vi "Three part tester.vi"() -> ()   [LabVIEW 2009]
uses:
  <vilib>/Instr/_visa.llb/VISA Configure Serial Port (Instr).vi
panel:
  out "Cluster Display":T1
  out "Cluster 2 Display":T2
  in  "Stop":bool
  out "decimal integer string 2":string
  out "number 2":u8 format="%b"
  in  "Yellow Guitar LED":bool
  in  "Green Guitar LED":bool
  in  "Red Guitar LED":bool
  in  "Blue Guitar LED":bool
  in  "Orange Guitar LED":bool
  in  "Orange Bass LED":bool
  in  "Yellow Bass LED":bool
  in  "Green Bass LED":bool
  in  "Red Bass LED":bool
  in  "Blue Bass LED":bool
  in  "Red Drum":bool
  in  "GreenDrum":bool
  in  "VISA resource name":refnum<visa-resource-name>
  out "number":u8 format="%b"
  out "decimal integer string":string
  in  "Yellow Drum":bool
  in  "Blue Drum":bool
  # "Drums"
  # "Bass"
  # "Guitar"
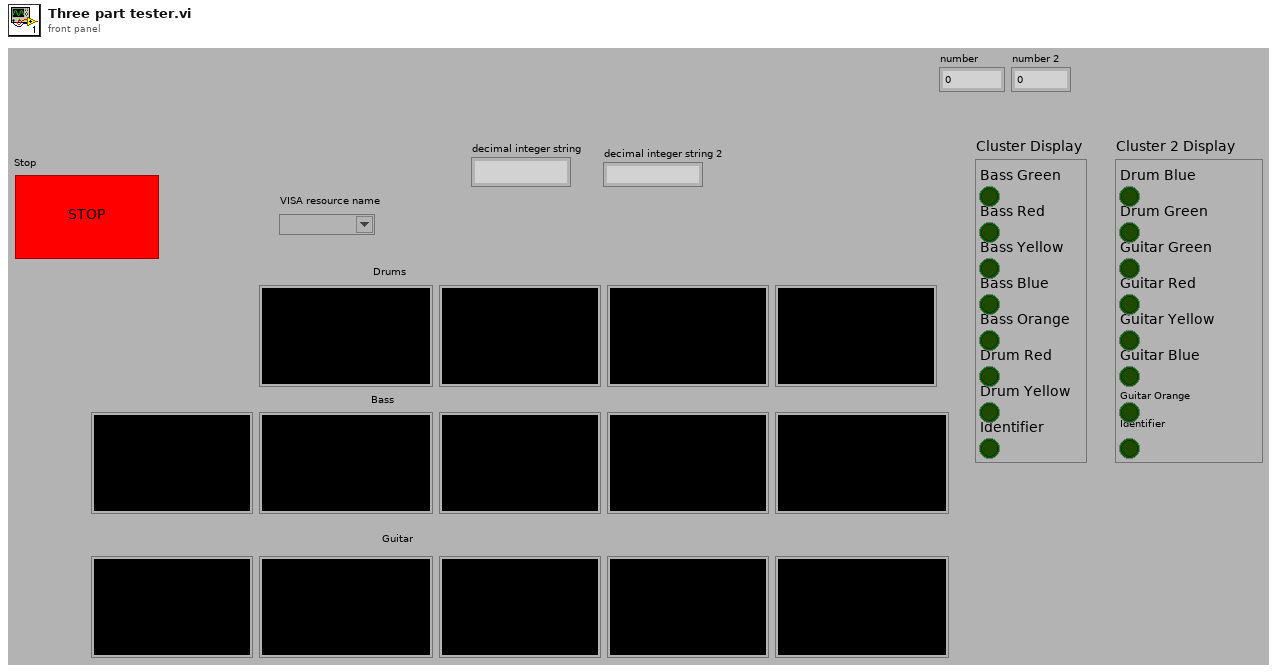
[diagram p1: front panel]
types:
  T1 = cluster{"Bass Green":bool, "Bass Red":bool, "Bass Yellow":bool, "Bass Blue":bool, "Bass Orange":bool, "Drum Red":bool, "Drum Yellow ":bool, "Identifier":bool}
  T2 = cluster{"Drum Blue":bool, "Drum Green":bool, "Guitar Green":bool, "Guitar Red":bool, "Guitar Yellow":bool, "Guitar Blue":bool, "Guitar Orange":bool, "Identifier":bool}
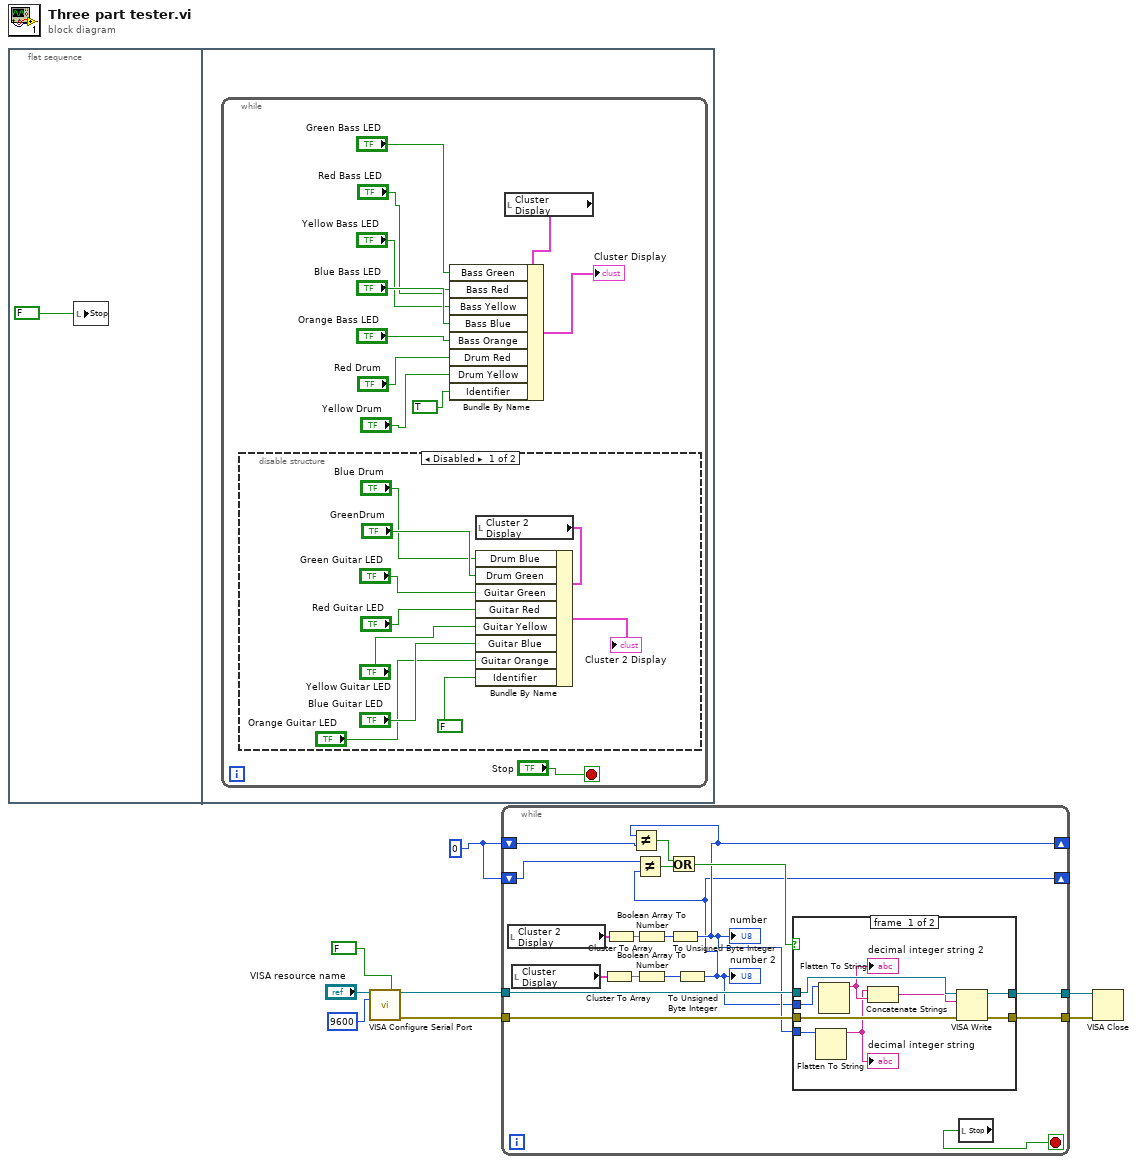
[diagram p0: block diagram]
diagram:
  w1 = u8 0
  n1 = flat-sequence {
    frame #0 {
      n2 = local write "Stop"(FALSE ("Stop 2")) -> ()
    }
    frame #1 {
      n3 = while {
        stop <- "Stop" stop-if-true
        n4 = disable-structure shown="Disabled" {
          frame #0 {
            n5 = local read "Cluster 2 Display"() -> (w29:T2)
            n6 = Bundle By Name(cluster=w29, "Drum Blue"="Blue Drum", "Drum Green"="GreenDrum", "Guitar Green"="Green Guitar LED", "Guitar Red"="Red Guitar LED", "Guitar Yellow"="Yellow Guitar LED", "Guitar Blue"="Blue Guitar LED", "Guitar Orange"="Orange Guitar LED", "Identifier"=FALSE ("element")) -> (→"Cluster 2 Display":T2)
          }
          frame #1 {
          }
        }
        n7 = local read "Cluster Display"() -> (w19:T1)
        n8 = Bundle By Name(cluster=w19, "Bass Green"="Green Bass LED", "Bass Red"="Red Bass LED", "Bass Yellow"="Yellow Bass LED", "Bass Blue"="Blue Bass LED", "Bass Orange"="Orange Bass LED", "Drum Red"="Red Drum", "Drum Yellow"="Yellow Drum", "Identifier"=TRUE ("element")) -> (→"Cluster Display":T1)
      }
    }
  }
  n9 = call-poly "VISA Configure Serial Port"("VISA resource name"="VISA resource name", "Enable Termination\nChar (T)"=FALSE ("Enable Termination\nChar (T)"), "baud rate (9600)"=u32 9600) -> ("VISA resource name out"=w8:refnum<visa-resource-name>, "error out"=w3:errorcluster)  [unwired: 11 in]
  n10 = while {
    tunnel: w8 -> [w48]
    tunnel: [w47] -> w7
    tunnel: w3 -> [w46]
    tunnel: [w45] -> w2
    shift-right: [w34] -> _
    shift-left: w1 -> [w33]
    shift-right: [w32] -> _
    shift-left: w1 -> [w31]
    stop <- w40 stop-if-true
    n11 = local read "Cluster 2 Display"() -> (w41:T2)
    n12 = local read "Cluster Display"() -> (w42:T1)
    n13 = Cluster To Array(cluster=w42) -> (array=w43:bool[])
    n14 = Cluster To Array(cluster=w41) -> (array=w44:bool[])
    n15 = Boolean Array To Number(Boolean array=w44) -> (number=w39:u32)
    n16 = Boolean Array To Number(Boolean array=w43) -> (number=w38:u32)
    n17 = To Unsigned Byte Integer(number=w39) -> (unsigned 8bit integer=w34:u8)
    "number" <- w34
    n18 = Not Equal?(x=w34, y=w33) -> (x != y?=w36:bool)
    n19 = To Unsigned Byte Integer(number=w38) -> (unsigned 8bit integer=w32:u8)
    "number 2" <- w32
    n20 = Not Equal?(x=w31, y=w32) -> (x != y?=w37:bool)
    n21 = Or(x=w36, y=w37) -> (x .or. y?=w35:bool)
    n22 = case shown="False" w35 {
      tunnel: w48 -> [w57 w59]
      tunnel: [w56 w59] -> w47
      tunnel: w34 -> [w50 _]
      tunnel: w46 -> [w55 w58]
      tunnel: [w54 w58] -> w45
      tunnel: w32 -> [w52 _]
      frame #0 {
        n23 = Flatten To String(anything=w50) -> (data string=w49:string)  [unwired: 3 in, 2 out]
        "decimal integer string" <- w49
        n24 = Flatten To String(anything=w52) -> (data string=w51:string)  [unwired: 3 in, 2 out]
        "decimal integer string 2" <- w51
        n25 = Concatenate Strings(w49, w51) -> (w53:string)
        n26 = VISA Write(VISA resource name=w57, write buffer=w53, error in (no error)=w55) -> (VISA resource name out=w56:refnum<visa-resource-name>, error out=w54:errorcluster)  [unwired: 1 out]
      }
      frame #1 {
      }
    }
    n27 = local read "Stop"() -> (w40:bool)
  }
  n28 = VISA Close(VISA resource name=w7, error in (no error)=w2) -> ()  [unwired: 1 out]
